vi "Grid_Scan_Stiching_dev.vi"() -> ()   [LabVIEW 2014]
uses:
  shared/CorrelImages (SubVI)Single.vi
  <userlib>/Nanonis Prog Interface V5/Nanonis Prog Interface.lvlib
panel:
  in  "Overlap (m)":dbl format="%#_6p"
  in  "Overlap (m)":cluster{"Width":sgl, "Height":sgl}
  in  "Pixels":i32 caption="Pixels/line"
  in  "Grid Coordinates":cluster{"Xc":sgl, "Yc":sgl} {"Yc" format="%.2p"; "Xc" format="%.2p"}
  out "floor(x/y)":i32
  out "yi":i32
  out "Grid Coordinates":dbl[][](array[numeric])
  in  "img delay (s)":u32=1
  in  "TipLift (m)":sgl format="%#_6p"
  out "timing":i32
  out "Grid Size":cluster{"Width":sgl, "Height":sgl}
  out "Angle (deg)":sgl format="%.2f"
  out "Size (m)":cluster{"Width":sgl, "Height":sgl} {"Height" format="%.2p"; "Width" format="%.2p"}
  out "Center coordinates (m)":cluster{"Xc":sgl, "Yc":sgl} {"Yc" format="%.2p"; "Xc" format="%.2p"}
  in  "# of Grids":i32=1 min=1 max=10
  in  "ref bias":dbl=-0.0012 format="%#_6p"
  out "DC active":bool
  out "Y drift":sgl
  out "X drift":sgl
  in  "Current":dbl=5e-11 format="%#_6p"
  in  "Bias":dbl=0.02 format="%#_6p"
  in  "Settling time (s)":dbl=0.7 format="%#_6p"
  in  "Channel index (0-23)":u8(ring) items=["Current"=0, "Z (m)"=14]
  in  "Img Speed":sgl=4.5e-08 format="%#_6p"
  in  "Img Bias (V) DC":sgl=1.0 format="%_2p"
  in  "Img Current":sgl=1e-10 format="%#_6p"
  in  "Drift correction Pixels":i32=128
  in  "Forward Speed":sgl=1.2e-09 format="%#_6p"
  in  "Backward Speed":sgl=8e-08 format="%#_6p"
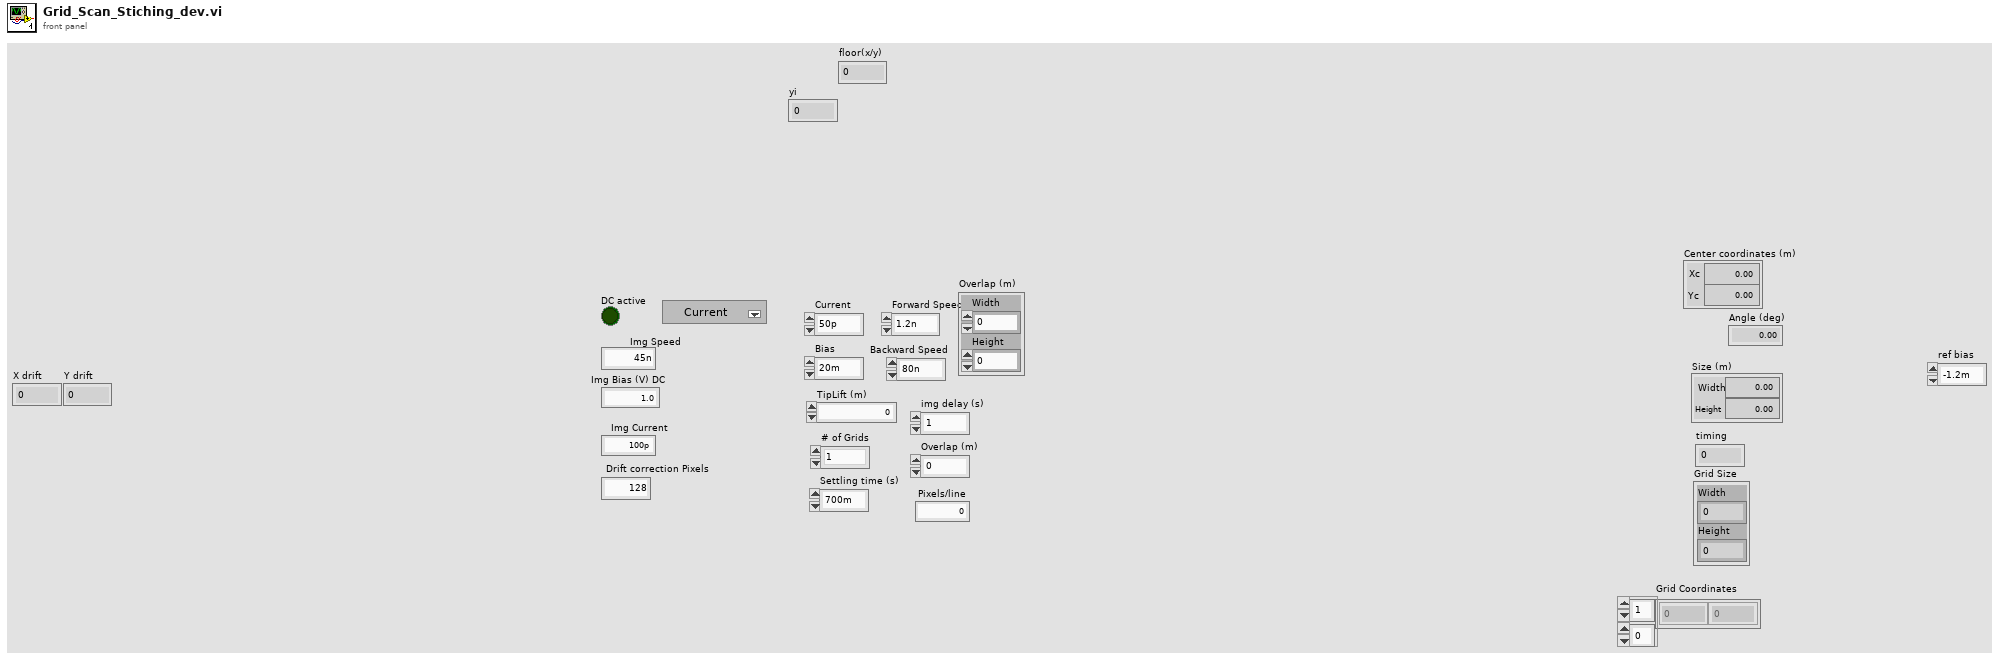
[diagram p1: front panel]
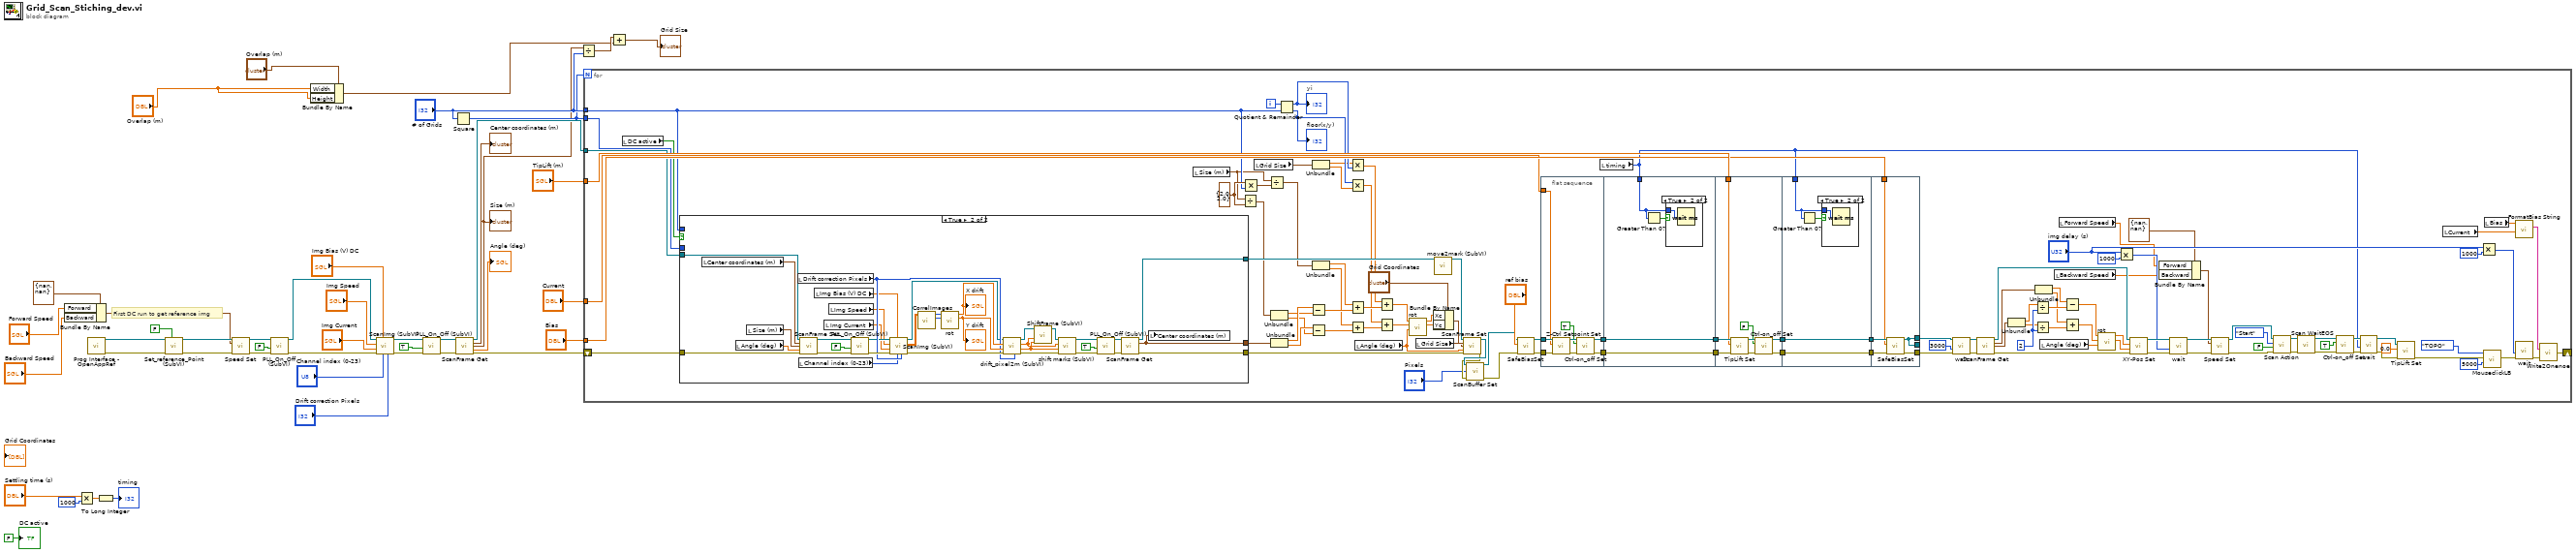
[diagram p0: block diagram]
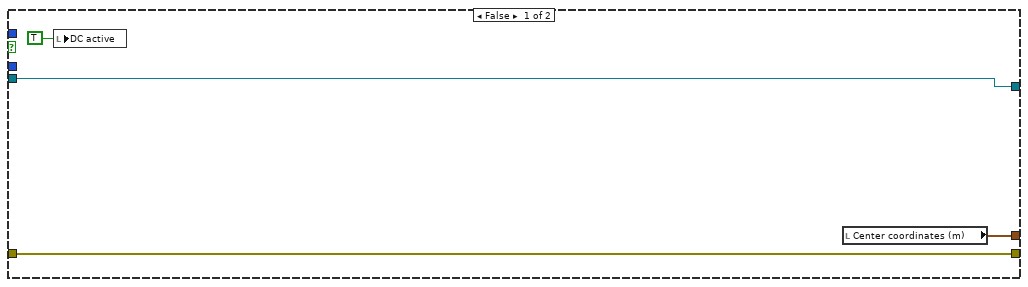
[diagram p2: hidden frame]
diagram:
  # "First DC run to get reference img"
  n1 = Bundle By Name(cluster=cluster{"Forward":sgl, "Backward":sgl} {"Forward"=nan, "Backward"=nan} ("Speed (m/s)"), "Forward"="Forward Speed", "Backward"="Backward Speed") -> (w37:cluster{"Forward":sgl, "Backward":sgl})
  n2 = Multiply(x="Settling time (s)", y=u32 1000) -> (x*y=w18:dbl)
  n3 = call <userlib>:"Prog Interface - OpenAppRef.vi"() -> ("Error out"=w43:errorcluster, "Application reference"=w44:refnum<vi>)  [unwired: 6 in]
  n4 = To Long Integer(number=w18) -> (32bit integer=→"timing":i32)
  n5 = call "Set_reference_Point (SubVI).vi"("Part of multigrid"=FALSE, "error in (no error)"=w43, "Application in"=w44) -> ("error out"=w39:errorcluster, "Application out"=w38:refnum<vi>)  [unwired: 7 in]
  n6 = call <userlib>:"Speed Set.vi"("Application ref in"=w38, "Speed (m/s)"=w37, "error in (no error)"=w39) -> ("Application ref out"=w34:refnum<vi>, "error out"=w35:errorcluster)  [unwired: 11 in]
  n7 = call "PLL_On_Off (SubVI).vi"("error in (no error)"=w35, "Output ON/OFF (F=OFF)"=FALSE, "Application in"=w34) -> ("error out"=w26:errorcluster, "Application out"=w27:refnum<vi>)  [unwired: 7 in]
  n8 = Bundle By Name(cluster="Overlap (m)", "Width"="Overlap (m)", "Height"="Overlap (m)") -> (w2:cluster{"Width":sgl, "Height":sgl})
  n9 = call "ScanImg (SubVI).vi"("pixel"="Drift correction Pixels", "Channel index (0-23)"="Channel index (0-23)", "Bias (V)"="Img Bias (V) DC", "error in (no error)"=w26, "Current"="Img Current", "Img Speed"="Img Speed", "Application in"=w27) -> ("error out"=w30:errorcluster, "Application out"=w31:refnum<vi>)  [unwired: 2 in, 1 out]
  n10 = call "PLL_On_Off (SubVI).vi"("error in (no error)"=w30, "Output ON/OFF (F=OFF)"=TRUE, "Application in"=w31) -> ("error out"=w22:errorcluster, "Application out"=w23:refnum<vi>)  [unwired: 7 in]
  n11 = Square(x="# of Grids") -> (x^2=w10:i32)
  n12 = call <userlib>:"ScanFrame Get.vi"("Application ref in"=w23, "error in (no error)"=w22) -> ("Application ref out"=w12:refnum<vi>, "Center coordinates (m)"=→"Center coordinates (m)":cluster{"Xc":sgl, "Yc":sgl}, "Size (m)"=w9:cluster{"Width":sgl, "Height":sgl}, "Angle (deg)"=→"Angle (deg)":sgl, "error out"=w6:errorcluster)  [unwired: 9 in]
  "Size (m)" <- w9
  n13 = Divide(x=w9, y="# of Grids") -> (x/y=w4:cluster{"Width":sgl, "Height":sgl})
  n14 = for {
    N: w10 -> [_]
    tunnel: "TipLift (m)" -> [w150]
    tunnel: "Bias" -> [w149]
    shift-right: [w56] -> _
    shift-left: w6 -> [w103]
    tunnel: "Current" -> [w105]
    tunnel: w12 -> [w101]
    tunnel: "# of Grids" -> [w96]
    tunnel: w10 -> [w100]
    i -> [w98]
    w97 = cluster{"Width":sgl, "Height":sgl} {"Width"=2.0, "Height"=2.0} ("y")
    w135 = 2
    n15 = local read "DC active"() -> (w60:bool)
    n16 = case shown="True" w60 {
      tunnel: [w164 w167] -> w104
      tunnel: w103 -> [w164 w174]
      tunnel: [w163 w175] -> w102
      tunnel: w101 -> [w163 w173]
      tunnel: w96 -> [_ _]
      tunnel: w100 -> [_ _]
      tunnel: [w162 w166] -> w83
      frame False {
        n17 = local write "DC active"(TRUE ("DC active")) -> ()
        n18 = local read "Center coordinates (m)"() -> (w162:cluster{"Xc":sgl, "Yc":sgl})
      }
      frame True {
        n19 = local read "Center coordinates (m)"() -> (w170:cluster{"Xc":sgl, "Yc":sgl})
        n20 = local read "Angle (deg)"() -> (w168:sgl)
        n21 = local read "Size (m)"() -> (w169:cluster{"Width":sgl, "Height":sgl})
        n22 = local read "Drift correction Pixels"() -> (w194:i32)
        n23 = local read "Channel index (0-23)"() -> (w189:u8)
        n24 = call <userlib>:"ScanFrame Set.vi"("Application ref in"=w173, "Center coordinates (m)"=w170, "Size (m)"=w169, "Angle (deg)"=w168, "error in (no error)"=w174) -> ("Application ref out"=w172:refnum<vi>, "error out"=w171:errorcluster)  [unwired: 9 in]
        n25 = local read "Img Bias (V) DC"() -> (w188:sgl)
        n26 = local read "Img Current"() -> (w187:sgl)
        n27 = local read "Img Speed"() -> (w186:sgl)
        n28 = call "PLL_On_Off (SubVI).vi"("error in (no error)"=w171, "Output ON/OFF (F=OFF)"=FALSE, "Application in"=w172) -> ("error out"=w199:errorcluster, "Application out"=w192:refnum<vi>)  [unwired: 7 in]
        n29 = call "ScanImg (SubVI).vi"("pixel"=w194, "Channel index (0-23)"=w189, "Bias (V)"=w188, "error in (no error)"=w199, "Current"=w187, "Img Speed"=w186, "Application in"=w192) -> ("error out"=w200:errorcluster, "Img"=w185:dbl[][], "Application out"=w191:refnum<vi>)  [unwired: 2 in]
        n30 = call-poly "CorrelImages.vi"("New Image"=w185) -> ("Y drift"=w197:i32, "X drift"=w195:i32)  [unwired: 7 in, 2 out]
        n31 = call "rot.vi"("y"=w197, "x"=w195) -> ("y'"=w198:sgl, "x'"=w196:sgl)  [unwired: 8 in]
        "X drift" <- w196
        "Y drift" <- w198
        n32 = call "drift_pixel2m (SubVI).vi"("Application in"=w191, "X drift"=w196, "Y drift"=w198, "error in"=w200, "Drift correction Pixels"=w194) -> ("Application out"=w190:refnum<vi>, "x drift"=w183:sgl, "y drift"=w182:sgl, "error out"=w181:errorcluster)  [unwired: 1 in]
        n33 = call "ShiftFrame (SubVI).vi"("Y shift"=w182, "X shift"=w183, "Application in"=w190) -> ("Application out"=w184:refnum<vi>)  [unwired: 8 in]
        n34 = call "shift marks (SubVI).vi"("error in (no error)"=w181, "y"=w182, "x"=w183, "Application in"=w184) -> ("error out"=w179:errorcluster, "Application out"=w180:refnum<vi>)  [unwired: 6 in]
        n35 = call "PLL_On_Off (SubVI).vi"("error in (no error)"=w179, "Output ON/OFF (F=OFF)"=TRUE, "Application in"=w180) -> ("error out"=w176:errorcluster, "Application out"=w177:refnum<vi>)  [unwired: 7 in]
        n36 = call <userlib>:"ScanFrame Get.vi"("Application ref in"=w177, "error in (no error)"=w176) -> ("Application ref out"=w175:refnum<vi>, "Center coordinates (m)"=w166:cluster{"Xc":sgl, "Yc":sgl}, "error out"=w167:errorcluster)  [unwired: 9 in, 2 out]
        n37 = local write "Center coordinates (m)"(w166) -> ()
      }
    }
    n38 = local read "Size (m)"() -> (w94:cluster{"Width":sgl, "Height":sgl})
    n39 = Divide(x=w94, y=w97) -> (x/y=w99:cluster{"Width":sgl, "Height":sgl})
    n40 = Multiply(x=w97, y=w96) -> (x*y=w95:cluster{"Width":sgl, "Height":sgl})
    n41 = local read "Grid Size"() -> (w69:cluster{"Width":sgl, "Height":sgl})
    n42 = Divide(x=w94, y=w95) -> (x/y=w93:cluster{"Width":sgl, "Height":sgl})
    n43 = Unbundle(w99) -> ("Width"=w89:sgl, "Height"=w87:sgl)
    n44 = Unbundle(w83) -> ("Xc"=w90:sgl, "Yc"=w88:sgl)
    n45 = Quotient & Remainder(x=w98, y=w96) -> (x-y*floor(x/y)=w91:i32, floor(x/y)=w92:i32)
    "yi" <- w91
    "floor(x/y)" <- w92
    n46 = Subtract(x=w90, y=w89) -> (x-y=w86:sgl)
    n47 = Subtract(x=w88, y=w87) -> (x-y=w85:sgl)
    n48 = Unbundle(w69) -> ("Width"=w68:sgl, "Height"=w67:sgl)
    n49 = Unbundle(w93) -> ("Width"=w71:sgl, "Height"=w70:sgl)
    n50 = Multiply(x=w68, y=w91) -> (x*y=w64:sgl)
    n51 = Multiply(x=w92, y=w67) -> (x*y=w61:sgl)
    n52 = Add(x=w71, y=w86) -> (x+y=w65:sgl)
    n53 = Add(x=w70, y=w85) -> (x+y=w62:sgl)
    n54 = local read "Angle (deg)"() -> (w80:sgl)
    n55 = Add(x=w64, y=w65) -> (x+y=w66:sgl)
    n56 = Add(x=w61, y=w62) -> (x+y=w63:sgl)
    n57 = call "rot.vi"("angle"=w80, "y"=w63, "x"=w66) -> ("y'"=w81:sgl, "x'"=w82:sgl)  [unwired: 7 in]
    n58 = local read "Grid Size"() -> (w113:cluster{"Width":sgl, "Height":sgl})
    n59 = Bundle By Name(cluster="Grid Coordinates", "Xc"=w82, "Yc"=w81) -> (w114:cluster{"Xc":sgl, "Yc":sgl})
    n60 = call "move2mark (SubVI).vi"("Application in"=w102) -> ("Application out"=w115:refnum<vi>)  [unwired: 10 in]
    n61 = call <userlib>:"ScanFrame Set.vi"("Application ref in"=w115, "Center coordinates (m)"=w114, "Size (m)"=w113, "Angle (deg)"=w80, "error in (no error)"=w104) -> ("Application ref out"=w49:refnum<vi>, "error out"=w46:errorcluster)  [unwired: 9 in]
    n62 = call <userlib>:"ScanBuffer Set.vi"("Application ref in"=w49, "Pixels"="Pixels", "error in (no error)"=w46) -> ("Application ref out"=w48:refnum<vi>, "error out"=w47:errorcluster)  [unwired: 11 in]
    n63 = call "SafeBiasSet.vi"("Application ref in"=w48, "Bias (V)"="ref bias", "error in (no error)"=w47) -> ("Application ref out"=w152:refnum<vi>, "Error out"=w153:errorcluster)  [unwired: 6 in]
    n64 = flat-sequence {
      tunnel: [w207] -> w161
      tunnel: [w204] -> w160
      tunnel: w152 -> [w203]
      tunnel: w153 -> [w202]
      tunnel: w105 -> [w201]
      tunnel: w161 -> [w212]
      tunnel: [w212] -> w159
      tunnel: w118 -> [w210]
      tunnel: [w209] -> w158
      tunnel: w160 -> [w209]
      tunnel: w159 -> [w221]
      tunnel: [w219] -> w157
      tunnel: w158 -> [w218]
      tunnel: [w216] -> w156
      tunnel: w150 -> [w214]
      tunnel: w157 -> [w225]
      tunnel: [w225] -> w155
      tunnel: [w223] -> w154
      tunnel: w156 -> [w223]
      tunnel: w118 -> [w222]
      tunnel: [w227] -> _
      tunnel: w155 -> [w231]
      tunnel: w154 -> [w230]
      tunnel: [w229] -> w117
      tunnel: w149 -> [w228]
      tunnel: [w227] -> w116
      frame #0 {
        n65 = call <userlib>:"Z-Ctrl Setpoint Set.vi"("error in (no error)"=w202, "Z Controller setpoint"=w201, "Application ref in"=w203) -> ("error out"=w205:errorcluster, "Application ref out"=w208:refnum<vi>)  [unwired: 7 in]
        n66 = call <userlib>:"Ctrl-on_off Set.vi"("error in (no error)"=w205, "Z Controller ON/OFF"=TRUE, "Application ref in"=w208) -> ("error out"=w204:errorcluster, "Application ref out"=w207:refnum<vi>)  [unwired: 7 in]
      }
      frame #1 {
        n67 = Greater Than 0?(x=w210) -> (x > 0?=w211:bool)
        n68 = case shown="True" w211 {
          tunnel: w210 -> [_ w213]
          frame False {
          }
          frame True {
            n69 = Wait (ms)(milliseconds to wait=w213) -> ()  [unwired: 1 out]
          }
        }
      }
      frame #2 {
        n70 = call <userlib>:"TipLift Set.vi"("error in (no error)"=w218, "TipLift (m)"=w214, "Application ref in"=w221) -> ("error out"=w217:errorcluster, "Application ref out"=w220:refnum<vi>)  [unwired: 7 in]
        n71 = call <userlib>:"Ctrl-on_off Set.vi"("error in (no error)"=w217, "Z Controller ON/OFF"=FALSE, "Application ref in"=w220) -> ("error out"=w216:errorcluster, "Application ref out"=w219:refnum<vi>)  [unwired: 7 in]
      }
      frame #3 {
        n72 = Greater Than 0?(x=w222) -> (x > 0?=w224:bool)
        n73 = case shown="True" w224 {
          tunnel: w222 -> [_ w226]
          frame False {
          }
          frame True {
            n74 = Wait (ms)(milliseconds to wait=w226) -> ()  [unwired: 1 out]
          }
        }
      }
      frame #4 {
        n75 = call "SafeBiasSet.vi"("Application ref in"=w231, "Bias (V)"=w228, "error in (no error)"=w230) -> ("Application ref out"=w227:refnum<vi>, "Error out"=w229:errorcluster)  [unwired: 6 in]
      }
    }
    n76 = local read "timing"() -> (w118:i32)
    n77 = call "wait.vi"("error in"=w117, "milliseconds to wait"=u32 3000 ("y"), "application reference in"=w116) -> ("error out"=w127:errorcluster, "application reference out"=w126:refnum<vi>)  [unwired: 7 in]
    n78 = call <userlib>:"ScanFrame Get.vi"("Application ref in"=w126, "error in (no error)"=w127) -> ("Application ref out"=w144:refnum<vi>, "Center coordinates (m)"=w130:cluster{"Xc":sgl, "Yc":sgl}, "Size (m)"=w131:cluster{"Width":sgl, "Height":sgl}, "error out"=w143:errorcluster)  [unwired: 9 in, 1 out]
    n79 = Unbundle(w131) -> ("Width"=w133:sgl, "Height"=w134:sgl)
    n80 = Divide(x=w133, y=w135) -> (x/y=w137:sgl)
    n81 = Divide(x=w134, y=w135) -> (x/y=w136:sgl)
    n82 = Unbundle(w130) -> ("Xc"=w138:sgl, "Yc"=w132:sgl)
    n83 = local read "Angle (deg)"() -> (w110:sgl)
    n84 = local read "Backward Speed"() -> (w73:sgl)
    n85 = local read "Forward Speed"() -> (w72:sgl)
    n86 = Subtract(x=w138, y=w137) -> (x-y=w112:sgl)
    n87 = Add(x=w132, y=w136) -> (x+y=w111:sgl)
    n88 = call "rot.vi"("angle"=w110, "y"=w111, "x"=w112) -> ("y'"=w108:sgl, "x'"=w109:sgl)  [unwired: 7 in]
    n89 = Multiply(x="img delay (s)", y=u32 1000) -> (x*y=w140:u32)
    n90 = call <userlib>:"XY-Pos Set.vi"("error in (no error)"=w143, "Y (m)"=w108, "X (m)"=w109, "Application ref in"=w144) -> ("error out"=w142:errorcluster, "Application ref out"=w141:refnum<vi>)  [unwired: 4 in]
    n91 = Bundle By Name(cluster=cluster{"Forward":sgl, "Backward":sgl} {"Forward"=nan, "Backward"=nan} ("Speed (m/s)"), "Forward"=w72, "Backward"=w73) -> (w74:cluster{"Forward":sgl, "Backward":sgl})
    n92 = call "wait.vi"("error in"=w142, "milliseconds to wait"=w140, "application reference in"=w141) -> ("error out"=w79:errorcluster, "application reference out"=w77:refnum<vi>)  [unwired: 7 in]
    n93 = call <userlib>:"Speed Set.vi"("Application ref in"=w77, "Speed (m/s)"=w74, "error in (no error)"=w79) -> ("Application ref out"=w76:refnum<vi>, "error out"=w78:errorcluster)  [unwired: 11 in]
    n94 = call <userlib>:"Scan Action.vi"("error in (no error)"=w78, "Direction: up/down (T=up)"=FALSE, "Scan action (Start)"=enum16{"Start", "Stop", "Pause", "Resume"}."Start", "Application ref in"=w76) -> ("error out"=w124:errorcluster, "Application ref out"=w125:refnum<vi>)  [unwired: 5 in]
    n95 = call <userlib>:"Scan WaitEOS.vi"("error in (no error)"=w124, "Application ref in"=w125) -> ("error out"=w106:errorcluster, "Application ref out"=w107:refnum<vi>)  [unwired: 5 in, 2 out]
    n96 = call <userlib>:"Ctrl-on_off Set.vi"("error in (no error)"=w106, "Z Controller ON/OFF"=TRUE, "Application ref in"=w107) -> ("error out"=w122:errorcluster, "Application ref out"=w120:refnum<vi>)  [unwired: 7 in]
    n97 = call "wait.vi"("error in"=w122, "milliseconds to wait"=w118, "application reference in"=w120) -> ("error out"=w121:errorcluster, "application reference out"=w119:refnum<vi>)  [unwired: 7 in]
    n98 = call <userlib>:"TipLift Set.vi"("error in (no error)"=w121, "TipLift (m)"=sgl 0.0, "Application ref in"=w119) -> ("error out"=w51:errorcluster)  [unwired: 7 in, 1 out]
    n99 = local read "Current"() -> (w54:dbl)
    n100 = Multiply(x="img delay (s)", y=u32 1000) -> (x*y=w145:u32)
    n101 = call "MouseclickLB.vi"("nMilliseconds"=5000, "error in (no error)"=w51, "Click"=enum16{"Header", "TOPO", "STS", "GRID"}."TOPO") -> ("error out"=w50:errorcluster)  [unwired: 8 in]
    n102 = local read "Bias"() -> (w55:dbl)
    n103 = call "FormatBias String.vi"("current"=w54, "bias"=w55) -> ("resulting string"=w58:string)  [unwired: 9 in]
    n104 = call "wait.vi"("error in"=w50, "milliseconds to wait"=w145) -> ("error out"=w57:errorcluster)  [unwired: 8 in, 1 out]
    n105 = call "Write2Onenoe.vi"("error in (no error)"=w57, "strSendText"=w58) -> ("error out"=w56:errorcluster)
  }
  n106 = Add(x=w4, y=w2) -> (x+y=→"Grid Size":cluster{"Width":sgl, "Height":sgl})
  "DC active" <- FALSE ("DC active")
